vi "testDmmBasic.vi"() -> ()   [LabVIEW 2023]
doc: "Illustrates how to use the Dmm Abstraction."
uses:
  Data/DmmTypes.ctl
  Data/DmmModes.ctl
  Multimeter.lvclass
  sweDmm.lvlib
panel:
  out "error out":errorcluster
  out "Result":dbl
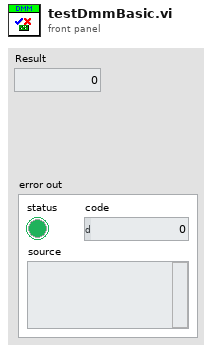
[diagram p1: front panel]
types:
  T1 = typedef "sweDmm.lvlib/DmmModes.ctl" = enum16{"VoltageDc", "VoltageAc", "CurrentDc", "CurrentAc", "Resistance2W"}
  T2 = typedef "sweDmm.lvlib/DmmTypes.ctl" = enum16{"Simulated", "DMM_NI", "DMM_Keysight"}
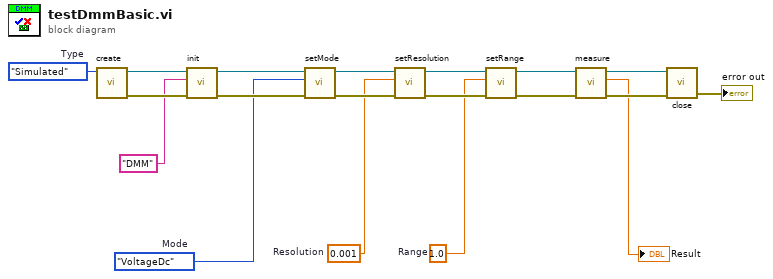
[diagram p0: block diagram]
diagram:
  w3 = 1.0  # Range
  w4 = 0.001  # Resolution
  w5 = DmmModes."VoltageDc"  # Mode
  w7 = DmmTypes."Simulated"  # Type
  n1 = call "create.vi"("Type"=w7) -> ("error out"=w18:errorcluster, "Multimeter.lvclass"=w19:refnum<class "Multimeter.lvclass">)  [unwired: 9 in]
  n2 = call-dynamic "init.vi"("error in (no error)"=w18, "Resource"="DMM", "Instrument in"=w19) -> ("error out"=w16:errorcluster, "Instrument out"=w17:refnum<class "Multimeter.lvclass">)  [unwired: 7 in]
  n3 = call-dynamic "setMode.vi"("error in (no error)"=w16, "Mode"=w5, "Multimeter in"=w17) -> ("error out"=w14:errorcluster, "Multimeter out"=w15:refnum<class "Multimeter.lvclass">)  [unwired: 7 in]
  n4 = call-dynamic "setResolution.vi"("error in (no error)"=w14, "Resolution"=w4, "Multimeter in"=w15) -> ("error out"=w12:errorcluster, "Multimeter out"=w13:refnum<class "Multimeter.lvclass">)  [unwired: 7 in]
  n5 = call-dynamic "setRange.vi"("error in (no error)"=w12, "Range"=w3, "Multimeter in"=w13) -> ("error out"=w10:errorcluster, "Multimeter out"=w11:refnum<class "Multimeter.lvclass">)  [unwired: 7 in]
  n6 = call-dynamic "measure.vi"("error in (no error)"=w10, "Multimeter in"=w11) -> ("error out"=w8:errorcluster, "Result"=→"Result":dbl, "Multimeter out"=w9:refnum<class "Multimeter.lvclass">)  [unwired: 7 in]
  n7 = call-dynamic "close.vi"("error in (no error)"=w8, "Instrument in"=w9) -> ("error out"=→"error out":errorcluster)  [unwired: 9 in]
